vi "LED亮度分析.vi"(0 "MyIndex":u8, 1 "亮阈值":i16=100, 2 "灭阈值":i16=100, 5 "地址":string="02", 9 "分析仪通道":T1(ring), 11 "error in (no error)":errorcluster caption="错误输入（无错误）") -> (4 "亮结果":string, 8 "灭结果":string, 10 "亮度":u16, 15 "error out":errorcluster caption="错误输出")   [LabVIEW 2015]
uses:
  <vilib>/Instr/_visa.llb/VISA Configure Serial Port (Instr).vi
panel:
  out "通道数据":u16[](array[numeric])
  out "Read":string
  out "Send":string
  # "R"
  # "G"
  # "B"
  # "i"
  # "H"
  # "S"
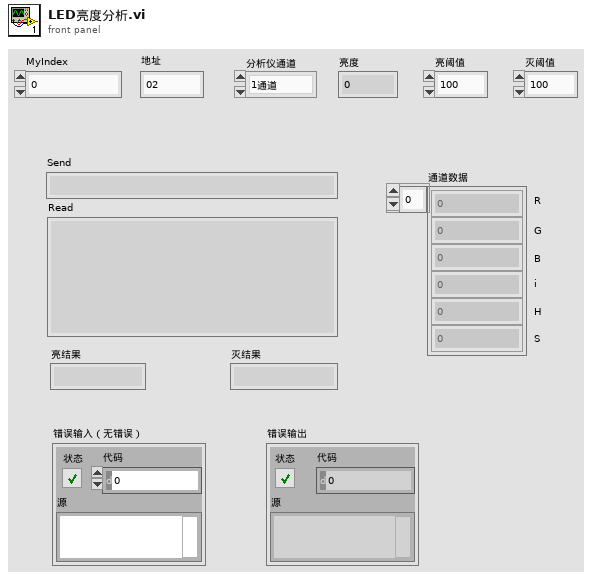
[diagram p1: front panel]
types:
  T1 = enum16{"1通道", "2通道", "3通道", "4通道", "5通道", "6通道", "7通道", "8通道", "9通道", "10通道", "11通道", "12通道", "13通道", "14通道", "15通道", "16通道", "17通道", "18通道", "19通道", "20通道", ""}
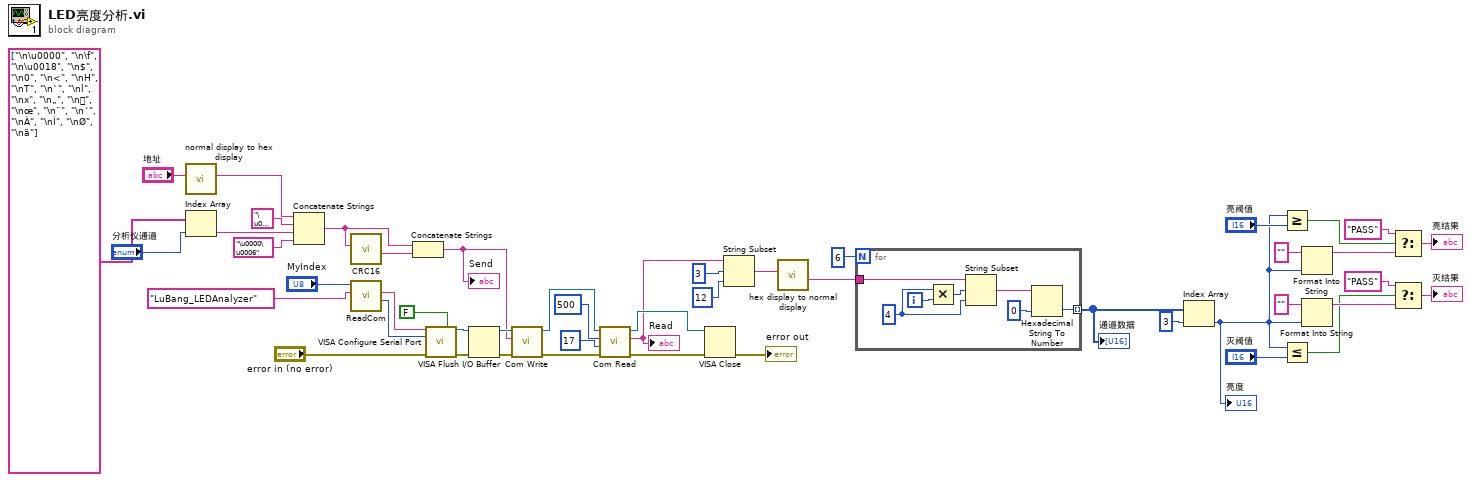
[diagram p0: block diagram]
diagram:
  n1 = call "normal display to hex display.vi"("Normal display"="地址") -> ("Hex display"=w41:string)  [unwired: 6 in]
  n2 = Index Array(array=string[] ["\n\u0000", "\n\f", "\n\u0018", "\n$", "\n0", "\n<", "\nH", "\nT", "\n`", "\nl", "\nx", "\n„", "\n", "\nœ", "\n¨", "\n´", "\nÀ", "\nÌ", "\nØ", "\nä"], index="分析仪通道") -> (element=w37:string)
  n3 = Concatenate Strings(w41, "\u0003", w37, "\u0000\u0006") -> (w45:string)
  n4 = call "CRC16.vi"("输入字符串"=w45) -> ("CRC16(String)"=w44:string)  [unwired: 9 in, 1 out]
  n5 = call "ReadCom.vi"("仪器名称"="LuBang_LEDAnalyzer", "MyIndex"="MyIndex") -> ("Baudrate"=w1:i32, "COM"=w2:string)  [unwired: 7 in, 1 out]
  n6 = Concatenate Strings(w45, w44) -> (w33:string)
  "Send" <- w33
  n7 = call-poly "VISA Configure Serial Port"("VISA resource name"=w2, "Enable Termination\nChar (T)"=FALSE ("Enable Termination\nChar (T)"), "baud rate (9600)"=w1, "error in (no error)"="error in (no error)") -> ("VISA resource name out"=w46:refnum<visa-resource-name>, "error out"=w47:errorcluster)  [unwired: 10 in]
  n8 = VISA Flush I/O Buffer(VISA resource name=w46, error in (no error)=w47) -> (VISA resource name out=w35:refnum<visa-resource-name>, error out=w34:errorcluster)  [unwired: 1 in]
  n9 = call "Com Write.vi"("错误输入（无错误）"=w34, "Wbuff"=w33, "VISA In"=w35) -> ("错误输出"=w32:errorcluster, "VISA Out"=w31:refnum<visa-resource-name>)  [unwired: 7 in]
  n10 = call "Com Read.vi"("错误输入（无错误）"=w32, "num"=u32 17, "超时"=u32 500, "VISA In"=w31) -> ("错误输出"=w27:errorcluster, "buff"=w26:string, "VISA Out"=w28:refnum<visa-resource-name>)  [unwired: 5 in]
  "Read" <- w26
  n11 = VISA Close(VISA resource name=w28, error in (no error)=w27) -> (error out=→"error out":errorcluster)
  n12 = String Subset(string=w26, offset (0)=3 ("长度（剩余）"), length (rest)=12 ("长度（剩余）")) -> (substring=w23:string)
  n13 = call "hex display to normal display.vi"("Hex display"=w23) -> ("Normal display"=w22:string)  [unwired: 10 in]
  n14 = for {
    N: 6 -> [_]
    tunnel: w22 -> [w55]
    tunnel: [w50] -> w20 mode=indexing
    i -> [w54]
    w52 = 4
    n15 = Multiply(x=w52, y=w54) -> (x*y=w53:i32)
    n16 = String Subset(string=w55, offset (0)=w53, length (rest)=w52) -> (substring=w51:string)
    n17 = Hexadecimal String To Number(string=w51, default (0uL)=u16 0) -> (number=w50:u16)  [unwired: 1 in, 1 out]
  }
  "通道数据" <- w20
  n18 = Index Array(array=w20, index=3) -> (element=w5:u16)
  "亮度" <- w5
  n19 = Greater Or Equal?(x=w5, y="亮阈值") -> (x >= y?=w16:bool)
  n20 = Less Or Equal?(x=w5, y="灭阈值") -> (x <= y?=w8:bool)
  n21 = Format Into String(initial string="" ("初始字符串"), w5) -> (resulting string=w12:string)  [unwired: 2 in, 1 out]
  n22 = Format Into String(initial string="" ("初始字符串"), w5) -> (resulting string=w11:string)  [unwired: 2 in, 1 out]
  n23 = Select(t="PASS", s=w16, f=w12) -> (s? t:f=→"亮结果":string)
  n24 = Select(t="PASS", s=w8, f=w11) -> (s? t:f=→"灭结果":string)
